vi "WPI_DashboardRetrieve NetworkTables2.vi"(8 "Docked Window":bool, 11 "DB Main Ref":refnum<vi>) -> (3 "Strings":T1)   [LabVIEW 2017]
uses:
  <vilib>/Rock Robotics/WPI/Dashboard/WPI_DashboardNTL Header Type.ctl
  <vilib>/Rock Robotics/WPI/Dashboard/WPI_DashboardLogging Global.vi
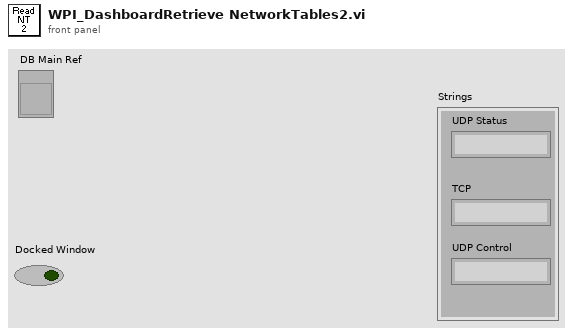
[diagram p1: front panel]
types:
  T1 = cluster{"UDP Status":string, "TCP":string, "UDP Control":string}
  T2 = typedef "WPI_DashboardNTL Header Type.ctl" = cluster{"Version":i32, "Duration (ms)":i32, "TimeStamp":timestamp, "Robot IP":string, "Displays":string[]}
  T3 = cluster{"Scale.Range:Minimum":dbl, dbl, "Scale.Range:Minimum":dbl, "Scale.Range:Minimum":dbl, "Scale.Range:Minimum":dbl}
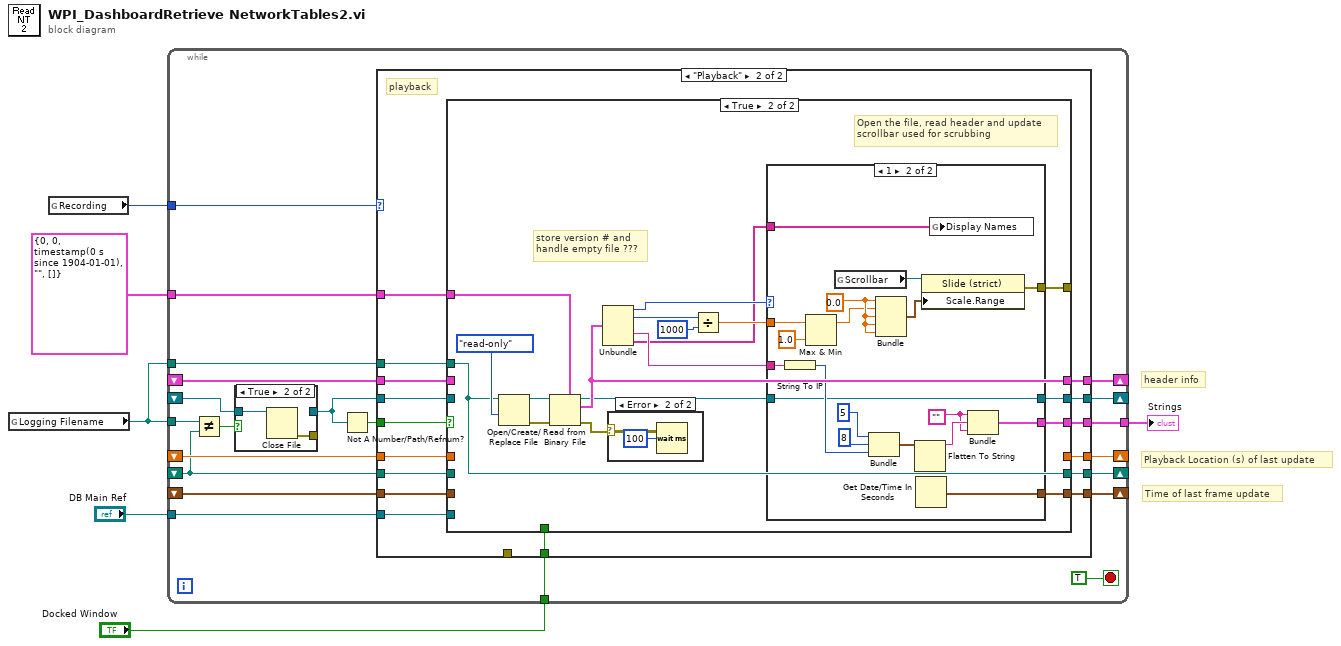
[diagram p0: block diagram]
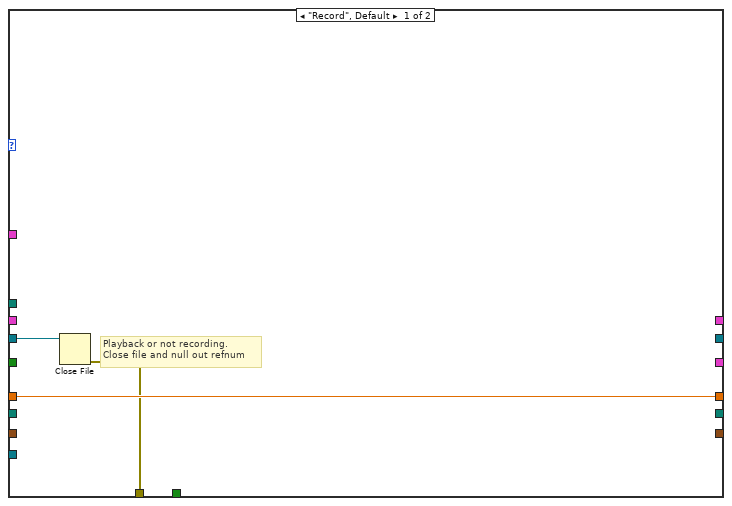
[diagram p3: hidden frame]
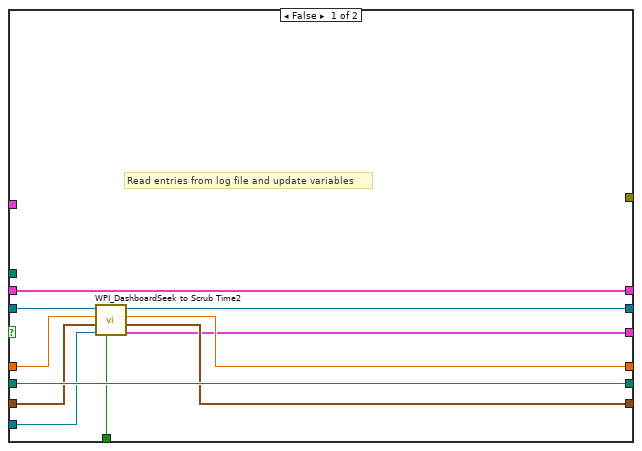
[diagram p4: hidden frame]
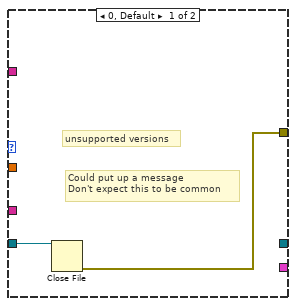
[diagram p5: hidden frame]
diagram:
  # "Time of last frame update"
  # "header info"
  # "Playback Location (s) of last update"
  n1 = global read "WPI_DashboardLogging Global.vi" "Logging Filename"() -> (w4:path)
  n2 = global read "WPI_DashboardLogging Global.vi" "Recording"() -> (w5:enum32{"Stop", "Record", "Playback"})
  n3 = while {
    shift-right: [w26] -> _
    shift-left: _ -> [w12]
    shift-right: [w24] -> _
    shift-left: _ -> [w23]
    shift-right: [w22] -> _
    shift-left: _ -> [w21]
    tunnel: T2 {"Version"=0, "Duration (ms)"=0, "TimeStamp"=timestamp(0 s since 1904-01-01), "Robot IP"="", "Displays"=[]} ("Header") -> [w20]
    shift-right: [w19] -> _
    shift-left: _ -> [w18]
    shift-right: [w16] -> _
    shift-left: _ -> [w15]
    tunnel: w5 -> [w9]
    tunnel: w4 -> [w17]
    tunnel: w4 -> [w11]
    tunnel: [w10] -> w1
    tunnel: "DB Main Ref" -> [w8]
    tunnel: "Docked Window" -> [w7]
    stop <- TRUE stop-if-true
    n4 = Not Equal?(x=w17, y=w15) -> (x != y?=w14:bool)
    n5 = case shown="True" w14 {
      tunnel: [w28 _] -> w13
      tunnel: w12 -> [w28 w30]
      tunnel: [_ w29] -> _
      frame False {
      }
      frame True {
        n6 = Close File(refnum=w30) -> (error out=w29:errorcluster)  [unwired: 1 in, 1 out]
      }
    }
    n7 = Not A Number/Path/Refnum?(number/path/refnum=w13) -> (NaN/Path/Refnum?=w25:bool)
    n8 = case shown="\"Playback\"" w9 {
      tunnel: [_ w49] -> w26
      tunnel: w13 -> [w33 w48]
      tunnel: w25 -> [_ w47]
      tunnel: [w32 w46] -> w24
      tunnel: w23 -> [w32 w45]
      tunnel: [_ w44] -> w22
      tunnel: w21 -> [_ w43]
      tunnel: w20 -> [_ w42]
      tunnel: [_ w41] -> w19
      tunnel: w18 -> [_ w40]
      tunnel: [_ w39] -> w16
      tunnel: w15 -> [_ w38]
      tunnel: w11 -> [_ w37]
      tunnel: [w31 _] -> _
      tunnel: [_ w36] -> w10
      tunnel: w8 -> [_ w35]
      tunnel: w7 -> [_ w34]
      frame "Record", Default {
        # "Playback or not recording.\nClose file and null out refnum"
        n9 = Close File(refnum=w33) -> (error out=w31:errorcluster)  [unwired: 1 in, 1 out]
      }
      frame "Playback" {
        # "playback"
        n10 = case shown="True" w47 {
          tunnel: [w53 w62] -> w49
          tunnel: w48 -> [w58 _]
          tunnel: [w52 _] -> w46
          tunnel: w45 -> [w57 _]
          tunnel: [w60 w75] -> w44
          tunnel: w43 -> [w60 _]
          tunnel: w42 -> [_ w74]
          tunnel: [w51 w71] -> w41
          tunnel: w40 -> [w56 _]
          tunnel: [w59 w70] -> w39
          tunnel: w38 -> [w59 _]
          tunnel: w37 -> [_ w70]
          tunnel: [_ w68] -> _
          tunnel: [w50 w65] -> w36
          tunnel: w35 -> [w55 _]
          tunnel: w34 -> [w54 _]
          frame False {
            # "Read entries from log file and update variables"
            n11 = call <vilib>:"WPI_DashboardSeek to Scrub Time2.vi"("Docked Window"=w54, "VI Refnum"=w55, "latest update tick"=w56, "TimeOffset (s)"=w57, "Byte Stream File in"=w58) -> ("Strings"=w50:T1, "ms tick out"=w51:timestamp, "TimeOffset (s) out"=w52:dbl, "Byte Stream File out"=w53:refnum<file>)  [unwired: 3 in]
          }
          frame True {
            # "store version # and\nhandle empty file ???"
            # "Open the file, read header and update\nscrollbar used for scrubbing"
            n12 = Open/Create/Replace File(file path (use dialog)=w70, access (0:read/write)=enum16{"read/write", "read-only", "write-only"}."read-only") -> (refnum out=w77:refnum<file>, error out=w76:errorcluster)  [unwired: 4 in, 1 out]
            n13 = Read from Binary File(5:w74, 8:w76, 11:w77) -> (0:w67:errorcluster, 2:w75:T2, 3:w63:refnum<file>)  [unwired: 3 in, 1 out]
            n14 = Unbundle(w75) -> ("Version"=w64:i32, "Duration (ms)"=w73:i32, "Robot IP"=w66:string, "Displays"=w61:string[])  [unwired: 1 out]
            n15 = case shown="Error" w67 {
              frame No Error {
              }
              frame Error {
                n16 = Wait (ms)(milliseconds to wait=u32 100) -> ()  [unwired: 1 out]
              }
            }
            n17 = Divide(x=w73, y=1000) -> (x/y=w69:dbl)
            n18 = case shown="1" w64 {
              tunnel: [_ w97] -> w71
              tunnel: w69 -> [_ w95]
              tunnel: [w79 w91] -> w68
              tunnel: w66 -> [_ w90]
              tunnel: [_ w83] -> w65
              tunnel: w63 -> [w80 w82]
              tunnel: [_ w82] -> w62
              tunnel: w61 -> [_ w81]
              frame 0, Default {
                # "Could put up a message\nDon't expect this to be common"
                # "unsupported versions"
                n19 = Close File(refnum=w80) -> (error out=w79:errorcluster)  [unwired: 1 in, 1 out]
              }
              frame 1 {
                w84 = ""
                w93 = 0.0 ("Scale.Range:Minimum")
                n20 = String To IP(1:w90) -> (0:w86:u32)
                n21 = Max & Min(x=w95, y=1.0 ("Scale.Range:Minimum")) -> (max(x,y)=w92:dbl)  [unwired: 1 out]
                n22 = global read "WPI_DashboardLogging Global.vi" "Scrollbar"() -> (w98:refnum<vi>)
                n23 = Bundle("index"=u16 5, "index"=u8 8, w86) -> (w88:cluster{"index":u16, "index":u8, u32})  [unwired: 1 in]
                n24 = Bundle("Scale.Range:Minimum"=w93, w92, "Scale.Range:Minimum"=w93, "Scale.Range:Minimum"=w93, "Scale.Range:Minimum"=w93) -> (w94:T3)  [unwired: 1 in]
                n25 = Flatten To String(anything=w88) -> (data string=w85:string)  [unwired: 3 in, 2 out]
                n26 = Get Date/Time In Seconds() -> (seconds since 1Jan1904=w97:timestamp)
                n27 = property class="Slide (strict)"(reference=w98, "Scale.Range"=w94) -> (error out=w91:errorcluster)  [unwired: 1 in, 1 out]
                n28 = global write "WPI_DashboardLogging Global.vi" "Display Names"(w81) -> ()
                n29 = Bundle(w84, "data string"=w85, w84) -> (w83:cluster{string, "data string":string, string})  [unwired: 1 in]
              }
            }
          }
        }
      }
    }
  }
  "Strings" <- w1
